vi "ATM_UpdateFile.vi"(0 "Balance":dbl) -> ()   [LabVIEW 2020]
panel:
  out "error out":errorcluster
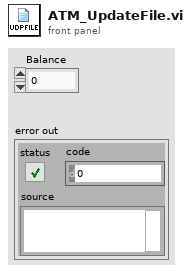
[diagram p1: front panel]
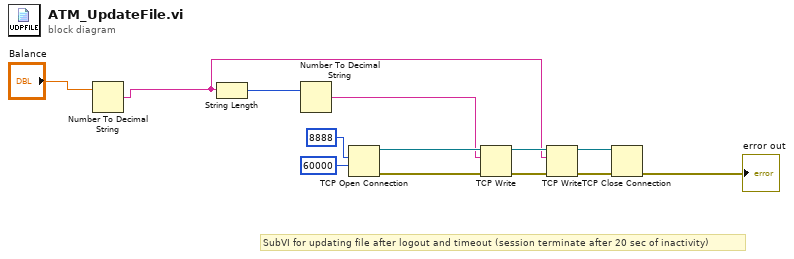
[diagram p0: block diagram]
diagram:
  # "SubVI for updating file after logout and timeout (session terminate after 20 sec of inactivity)"
  n1 = Number To Decimal String(number="Balance") -> (decimal integer string=w3:string)  [unwired: 1 in]
  n2 = String Length(string=w3) -> (length=w1:i32)
  n3 = Number To Decimal String(number=w1) -> (decimal integer string=w5:string)  [unwired: 1 in]
  n4 = TCP Open Connection(remote port or service name=u16 8888, timeout ms (60000)=60000) -> (connection ID=w11:refnum<k5>, error out=w8:errorcluster)  [unwired: 3 in]
  n5 = TCP Write(connection ID=w11, data in=w5, error in (no error)=w8) -> (connection ID out=w12:refnum<k5>, error out=w7:errorcluster)  [unwired: 1 in, 1 out]
  n6 = TCP Write(connection ID=w12, data in=w3, error in (no error)=w7) -> (connection ID out=w13:refnum<k5>, error out=w6:errorcluster)  [unwired: 1 in, 1 out]
  n7 = TCP Close Connection(connection ID=w13, error in (no error)=w6) -> (error out=→"error out":errorcluster)  [unwired: 1 in, 1 out]
